vi "Climber Global.vi"() -> ()   [LabVIEW 2019]
panel:
  out "Manual Climber":bool
  in  "Climb Speed":dbl
  in  "Level Climber":dbl
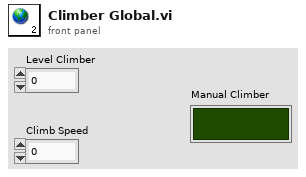
[diagram p1: front panel]
diagram:
